vi "Create.vi"(8 "error in (no error)":errorcluster, 11 "CIFPlugin in":refnum<class "Template_Plugin.lvclass">) -> (0 "error out":errorcluster, 3 "CIFPlugin out":refnum<class "Template_Plugin.lvclass">)   [LabVIEW 2021, in "Template_Plugin.lvclass"]
uses:
  Template_Plugin.lvclass
  C:/Program Files/National Instruments/LabVIEW 2021/vi.lib/CIF Foundation/CIF Core/CIFCore/Class/CIFCorePlugin.lvclass
  <vilib>/CIF Foundation/CIF Channels Core/CIFChannels/CIFChannels.lvclass
  Common/Template_Common.lvlib
  <vilib>/CIF Foundation/CIF Core/CIFCore/Class/CIFCorePlugin.lvclass
  <vilib>/CIF Foundation/CIF Core/CIFCore/Common/Typedef/Timing Overrides.ctl
  <vilib>/CIF Foundation/CIF Core/CIFCore/Common/CIFCoreCommon.lvlib
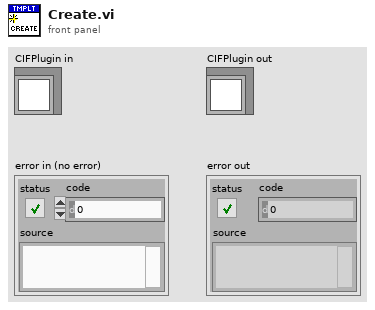
[diagram p1: front panel]
types:
  T1 = typedef "CIFCoreCommon.lvlib/Timing Overrides.ctl" = cluster{"Override Timing":bool, "Skip Sleep":bool, "Period (s)":dbl}
  T2 = typedef "ChannelRegistrar.lvlib/Channel Definition.ctl" = cluster{"Name":string, "Direction":T3, "Type":T4, "Custom Config Data":u8[]}
  T3 = typedef "ChannelCommon.lvlib/Direction.ctl" = enum8{"Publisher", "Subscriber"}
  T4 = typedef "ChannelRegistrar.lvlib/Registered Channel Types.ctl" = enum8{"Custom", "Double_Tag", "I64_Tag", "U64_Tag", "U8_FIFO", "CAN_FIFO", "L2Enet_FIFO", "DAQ_FIFO", "Universal_FIFO", "String_Tag"}
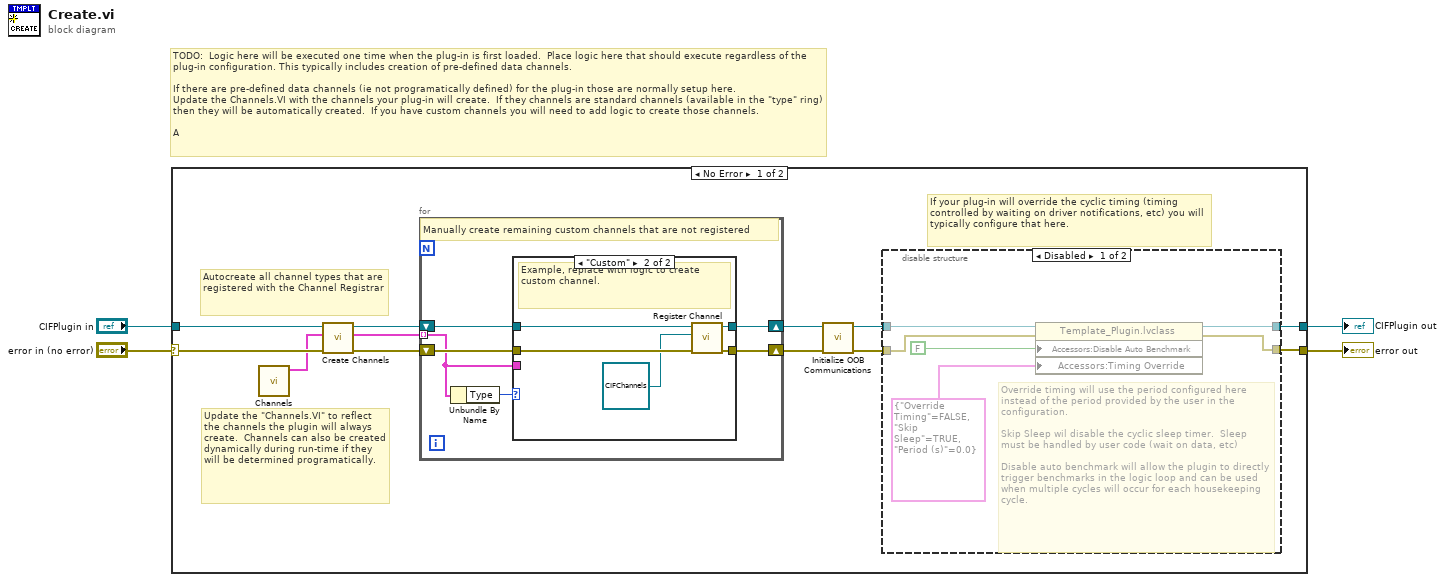
[diagram p0: block diagram]
diagram:
  # "TODO:  Logic here will be executed one time when the plug-in is first loaded.  Place logic here that should execute regardless of the plug-in configuration. This typically includes creation of pre-defined data channels.\n\nIf there are pre-defined data channels (ie not programatically defined) for the plug-in those are normally setup here.  \nUpdate the Channels.VI with the channels your plug-in will create.  If they channels are standard channels (available in the \"type\" ring) then they will be automatically created.  If you have custom channels you will need to add logic to create those channels.\n\nA"
  n1 = case shown="No Error" "error in (no error)" {
    selector: "error in (no error)" -> [w15 w39]
    tunnel: [w9 w39] -> w1
    tunnel: [w10 w38] -> w2
    tunnel: "CIFPlugin in" -> [w16 w38]
    frame No Error {
      # "If your plug-in will override the cyclic timing (timing controlled by waiting on driver notifications, etc) you will typically configure that here."
      # "Update the \"Channels.VI\" to reflect the channels the plugin will always create.  Channels can also be created dynamically during run-time if they will be determined programatically."
      # "Autocreate all channel types that are registered with the Channel Registrar"
      n2 = call "Channels.vi"() -> ("Channels to Create"=w14:T2[])  [unwired: 10 in, 1 out]
      n3 = call <vilib>:"Create Channels.vi"("error in (no error)"=w15, "Channels to Create in"=w14, "CIFCorePlugin in"=w16) -> ("error out"=w11:errorcluster, "Channels to Create out"=w13:T2[], "CIFCorePlugin out"=w12:refnum<class "Template_Plugin.lvclass">)  [unwired: 6 in]
      n4 = for {
        tunnel: w13 -> [w25] mode=indexing
        shift-right: [w28] -> w8
        shift-left: w12 -> [w30]
        shift-right: [w27] -> w7
        shift-left: w11 -> [w29]
        # "Manually create remaining custom channels that are not registered"
        n5 = Unbundle By Name(w25) -> ("Type"=w26:T4)
        n6 = case shown="\"Custom\"" w26 {
          tunnel: w30 -> [w32 w37]
          tunnel: w29 -> [w31 w36]
          tunnel: [w32 w35] -> w28
          tunnel: [w31 w34] -> w27
          tunnel: w25 -> [_ _]
          frame Default {
          }
          frame "Custom" {
            # "Example, replace with logic to create custom channel."
            n7 = call <vilib>:"Register Channel.vi"("error in (no error)"=w36, "Channel"=refnum<class "CIFChannels.lvclass"> refnum, "CIFCorePlugin in"=w37) -> ("error out"=w34:errorcluster, "CIFCorePlugin out"=w35:refnum<class "Template_Plugin.lvclass">)  [unwired: 7 in]
          }
        }
      }
      n8 = call "Initialize OOB Communications.vi"("error in (no error)"=w7, "CIFPlugin in"=w8) -> ("error out"=w5:errorcluster, "CIFPlugin out"=w6:refnum<class "Template_Plugin.lvclass">)  [unwired: 8 in]
      n9 = disable-structure shown="Disabled" {
        disable-tunnel: w6 -> [w22 w24]
        disable-tunnel: w5 -> [w21 w23]
        disable-tunnel: [w20 w24] -> w10
        disable-tunnel: [w19 w23] -> w9
        frame Disabled {
          # "Override timing will use the period configured here instead of the period provided by the user in the configuration.\n\nSkip Sleep wil disable the cyclic sleep timer.  Sleep must be handled by user code (wait on data, etc) \n\nDisable auto benchmark will allow the plugin to directly trigger benchmarks in the logic loop and can be used when multiple cycles will occur for each housekeeping cycle."
          n10 = property class="Template_Plugin.lvclass"(reference=w22, error in=w21, "Accessors:Disable Auto Benchmark"=FALSE ("Disable Auto Benchmark"), "Accessors:Timing Override"=T1 {"Override Timing"=FALSE, "Skip Sleep"=TRUE, "Period (s)"=0.0} ("Timing Override")) -> (reference out=w20:refnum<class "Template_Plugin.lvclass">, error out=w19:errorcluster)
        }
        frame Enabled {
        }
      }
    }
    frame Error {
    }
  }
  "CIFPlugin out" <- w2
  "error out" <- w1
